vi "timing_code.vi"   [LabVIEW 2017]
uses:
  <vilib>/myRIO/Common/Instrument Driver Framework/myRIO v1.0/DIO/typedefs/DIO Channels Enum.ctl
  <vilib>/myRIO/Common/Instrument Driver Framework/myRIO v1.0/DIO/typedefs/DIO Channels List.ctl
  <vilib>/myRIO/Common/Instrument Driver Framework/Utilities/typedefs/Generic FPGA Reference.ctl
  <vilib>/myRIO/Common/Instrument Driver Framework/Utilities/typedefs/myRIO v1.0 Reference.ctl
  <vilib>/myRIO/Common/Instrument Driver Framework/Utilities/typedefs/Hardware Version Enum.ctl
  <vilib>/myRIO/Common/Instrument Driver Framework/Utilities/typedefs/myRIO Generic Hardware Reference.ctl
  <vilib>/myRIO/Instrument Drivers/Onboard IO/DIO/typedefs/DIO Reference.ctl
  <vilib>/myRIO/Instrument Drivers/Onboard IO/DIO/DIO.lvlib
  <vilib>/myRIO/Instrument Drivers/Onboard IO/DIO/vis/Write.vi
  <vilib>/userdefined/High Color/nirio_resource_hc.ctl
  <vilib>/myRIO/Common/Instrument Driver Framework/myRIO v1.0/DIO/vis/myRIO v1.1 Open DIO.vi
  <vilib>/myRIO/Instrument Drivers/Onboard IO/DIO/vis/myRIO DIO Open.xnode
  <vilib>/myRIO/Common/Instrument Driver Framework/Utilities/vis/Is FPGA Ref Available.vi
  <vilib>/myRIO/Express VI/Onboard IO/DO/DO Express VI.xnode
types:
  T1 = typedef "DIO.lvlib/DIO Reference.ctl" = cluster{"myRIO Reference":T2, "DIO Channels List":T6}
  T2 = typedef "myRIO Generic Hardware Reference.ctl" = cluster{"myRIO Model":T3, "myRIO Hardware Reference":T4}
  T3 = typedef "Hardware Version Enum.ctl" = enum16{"Unknown", "myRIO-1900", "myRIO-1950", "roboRIO", "NI ELVIS RIO CM"}
  T4 = typedef "myRIO v1.0 Reference.ctl" = cluster{"Generic FPGA Reference":T5, "Allow multiple opens":bool}
  T5 = typedef "Generic FPGA Reference.ctl" = refnum<k20>
  T6 = typedef "DIO Channels List.ctl" = T7[]
  T7 = typedef "DIO Channels Enum.ctl" = enum16{"Not Connected", "C/DIO0", "C/DIO1", "C/DIO2", "C/DIO3", "C/DIO4", "C/DIO5", "C/DIO6", "C/DIO7", "A/DIO0", "A/DIO1", "A/DIO2", "A/DIO3", "A/DIO4", "A/DIO5", "A/DIO6", "A/DIO7", "A/DIO8", "A/DIO9", "A/DIO10", "A/DIO11", "A/DIO12", "A/DIO13", "A/DIO14", "A/DIO15", "B/DIO0", "B/DIO1", "B/DIO2", "B/DIO3", "B/DIO4", "B/DIO5", "B/DIO6", "B/DIO7", "B/DIO8", "B/DIO9", "B/DIO10", "B/DIO11", "B/DIO12", "B/DIO13", "B/DIO14", "B/DIO15", "LED0", "LED1", "LED2", "LED3", "Button0", "DIO/DIO0", "DIO/DIO1", "DIO/DIO2", "DIO/DIO3", "DIO/DIO4", "DIO/DIO5", "DIO/DIO6", "DIO/DIO7", "DIO/DIO8", "DIO/DIO9", "SPI/CS0", "SPI/CS1", "SPI/CS2", "SPI/CS3", "LED RADIO (Green)", "LED RADIO (Red)", "LED COMM (Green)", "LED COMM (Red)", "LED MODE (Green)", "LED MODE (Red)"}
  T8 = typedef "nirio_resource_hc.ctl" = tag
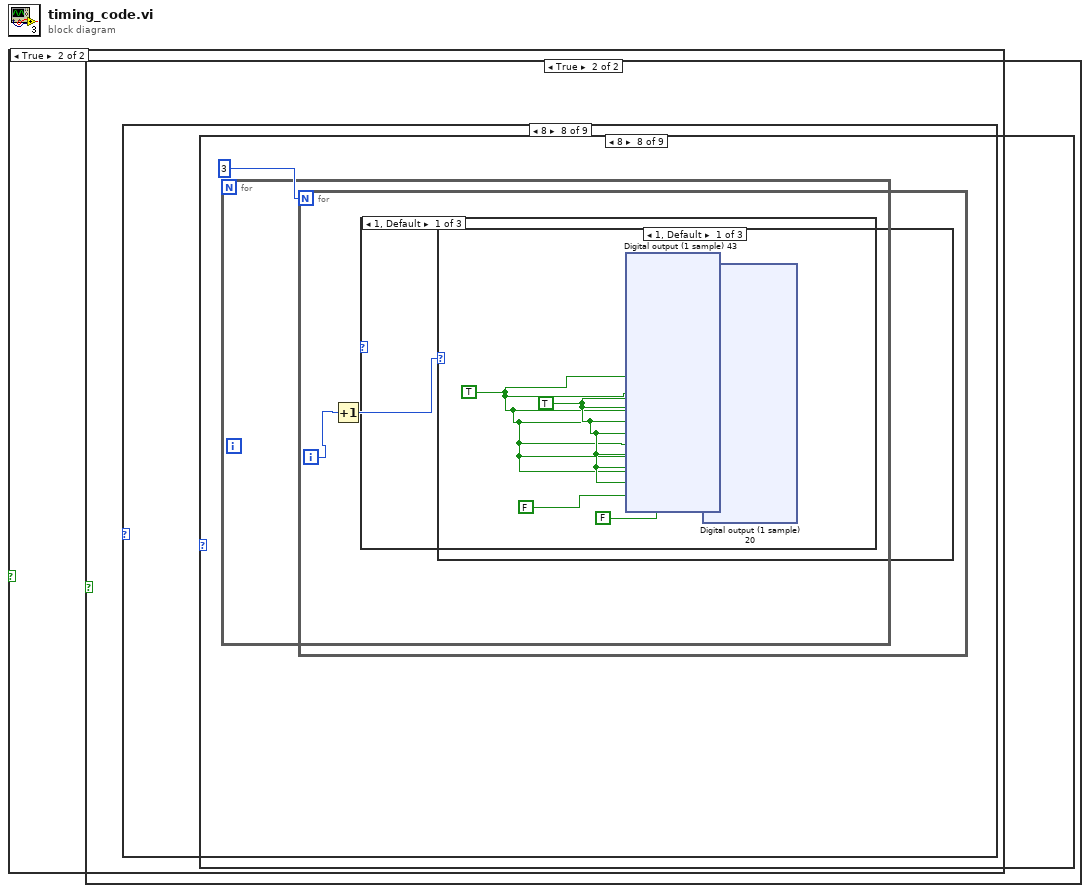
[diagram p0: block diagram]
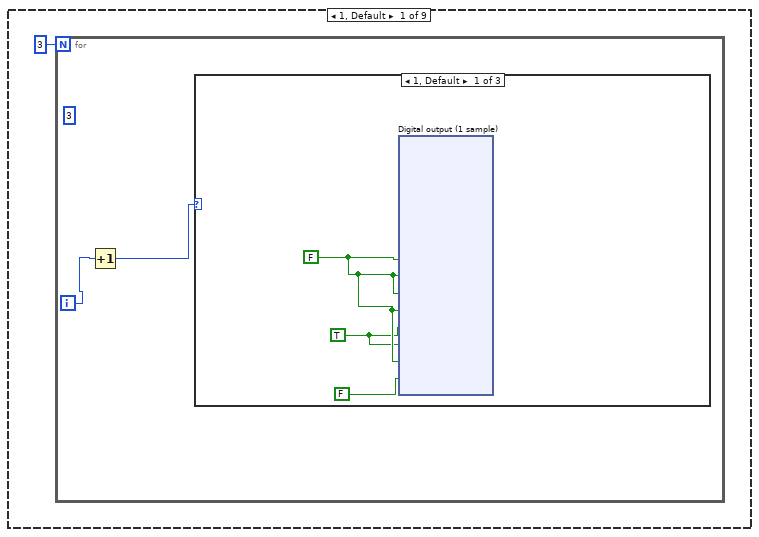
[diagram p3: hidden frame]
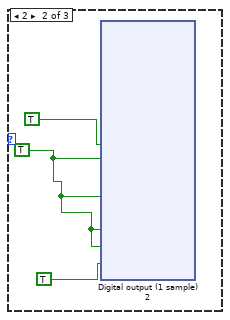
[diagram p4: hidden frame]
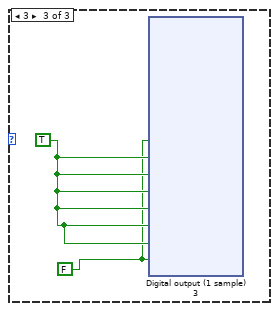
[diagram p5: hidden frame]
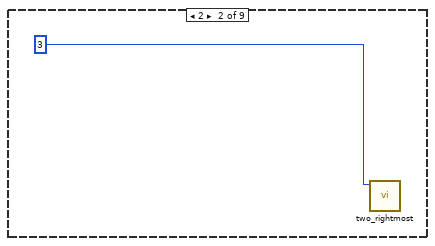
[diagram p6: hidden frame]
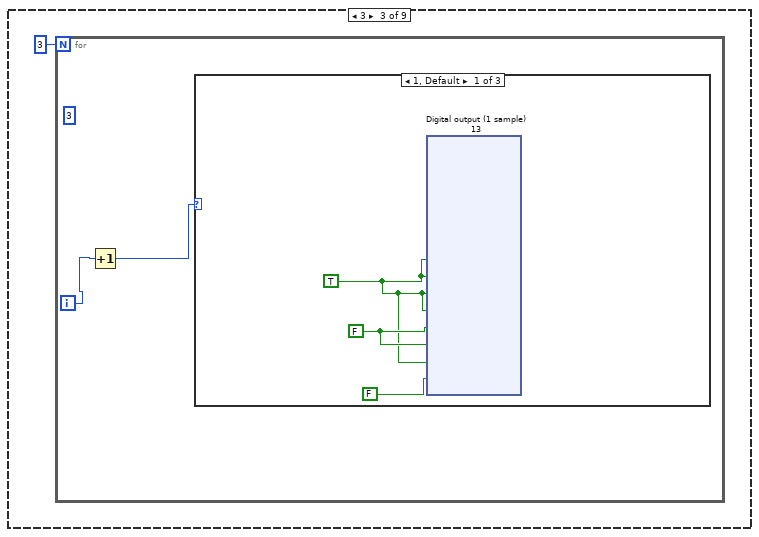
[diagram p7: hidden frame]
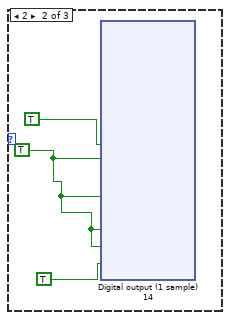
[diagram p8: hidden frame]
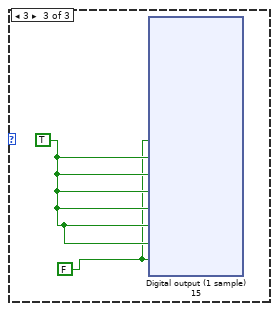
[diagram p9: hidden frame]
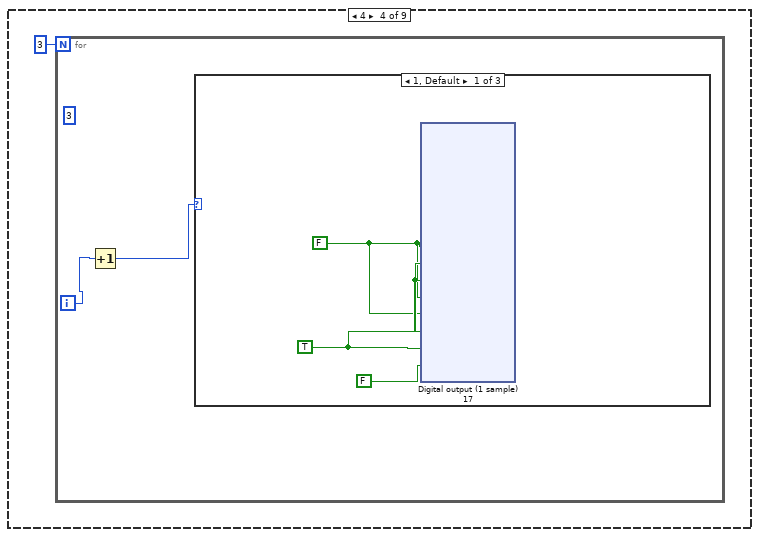
[diagram p10: hidden frame]
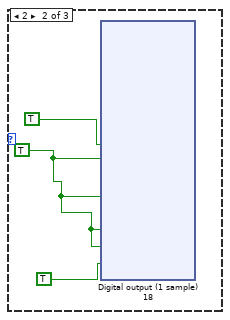
[diagram p11: hidden frame]
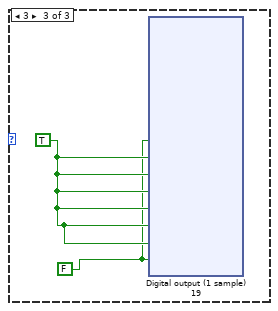
[diagram p12: hidden frame]
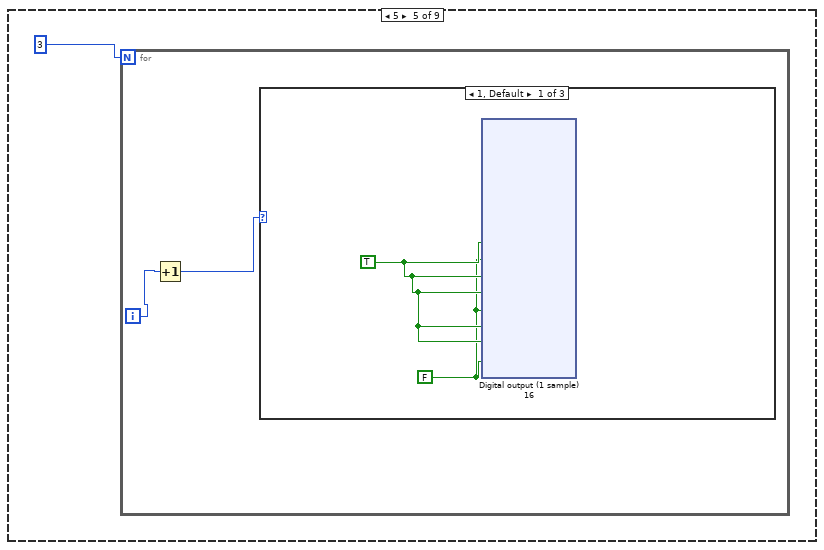
[diagram p13: hidden frame]
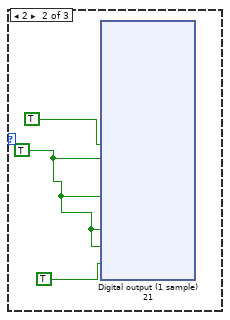
[diagram p14: hidden frame]
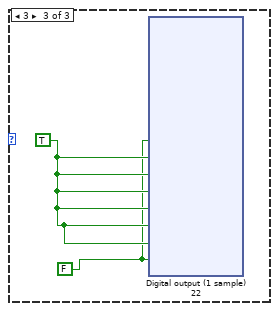
[diagram p15: hidden frame]
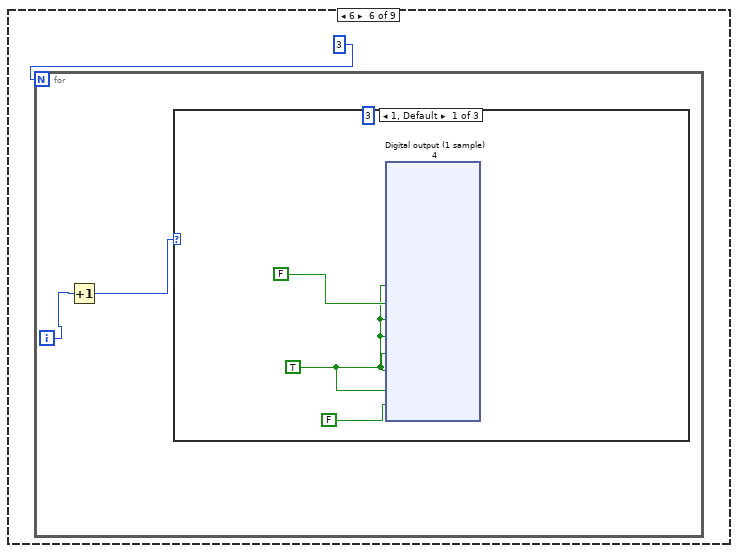
[diagram p16: hidden frame]
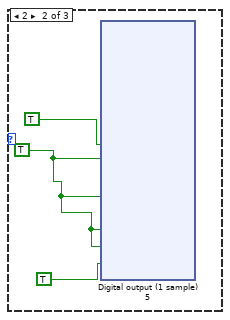
[diagram p17: hidden frame]
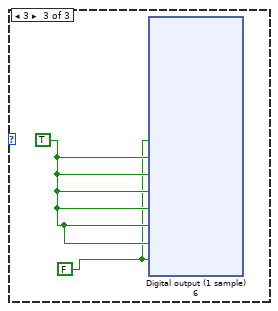
[diagram p18: hidden frame]
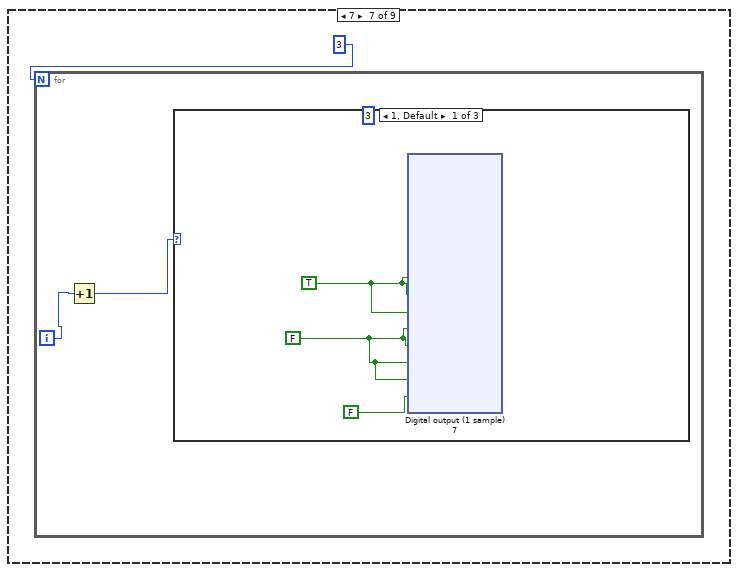
[diagram p19: hidden frame]
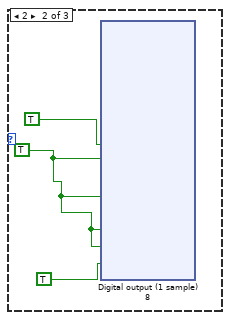
[diagram p20: hidden frame]
diagram:
  n1 = case shown="True" {
    selector: _ -> [_ _]
    frame False {
    }
    frame True {
      n2 = case shown="8" {
        selector: _ -> [_ _ _ _ _ _ _ _ _]
        frame 1, Default {
          (unwired) 3
          n3 = for {
            N: 3 -> [_]
            i -> [w3]
            n4 = Increment(x=w3) -> (x+1=w2:i32)
            n5 = case shown="1, Default" w2 {
              frame 1, Default {
                w4 = TRUE
                w5 = FALSE
                n6 = xnode "Digital output (1 sample)"("A/DIO0 (Pin 11)"=w5, "A/DIO1 (Pin 13)"=w5, "A/DIO2 (Pin 15)"=w5, "A/DIO3 (Pin 17)"=w5, "A/DIO4 (Pin 19)"=w4, "A/DIO5 (Pin 21)"=w4, "A/DIO6 (Pin 23)"=w5, "A/DIO7 (Pin 25)"=FALSE) -> ()  [unwired: 1 in, 1 out]
              }
              frame 2 {
                w49 = TRUE
                n7 = xnode "Digital output (1 sample) 2"("A/DIO0 (Pin 11)"=TRUE, "A/DIO1 (Pin 13)"=w49, "A/DIO2 (Pin 15)"=w49, "A/DIO3 (Pin 17)"=w49, "A/DIO4 (Pin 19)"=w49, "A/DIO5 (Pin 21)"=w49, "A/DIO6 (Pin 23)"=w49, "A/DIO7 (Pin 25)"=TRUE) -> ()  [unwired: 1 in, 1 out]
              }
              frame 3 {
                w95 = TRUE
                w94 = FALSE
                n8 = xnode "Digital output (1 sample) 3"("A/DIO0 (Pin 11)"=w94, "A/DIO1 (Pin 13)"=w95, "A/DIO2 (Pin 15)"=w95, "A/DIO3 (Pin 17)"=w95, "A/DIO4 (Pin 19)"=w95, "A/DIO5 (Pin 21)"=w95, "A/DIO6 (Pin 23)"=w95, "A/DIO7 (Pin 25)"=w94) -> ()  [unwired: 1 in, 1 out]
              }
            }
          }
        }
        frame 2 {
          n9 = call "two_rightmost.vi"("Numeric"=3) -> ()  [unwired: 11 in]
        }
        frame 3 {
          (unwired) 3
          n10 = for {
            N: 3 -> [_]
            i -> [w141]
            n11 = Increment(x=w141) -> (x+1=w140:i32)
            n12 = case shown="1, Default" w140 {
              frame 1, Default {
                w143 = FALSE
                w142 = TRUE
                n13 = xnode "Digital output (1 sample) 13"("A/DIO0 (Pin 11)"=w142, "A/DIO1 (Pin 13)"=w142, "A/DIO2 (Pin 15)"=w142, "A/DIO3 (Pin 17)"=w142, "A/DIO4 (Pin 19)"=w143, "A/DIO5 (Pin 21)"=w143, "A/DIO6 (Pin 23)"=w142, "A/DIO7 (Pin 25)"=FALSE) -> ()  [unwired: 1 in, 1 out]
              }
              frame 2 {
                w187 = TRUE
                n14 = xnode "Digital output (1 sample) 14"("A/DIO0 (Pin 11)"=TRUE, "A/DIO1 (Pin 13)"=w187, "A/DIO2 (Pin 15)"=w187, "A/DIO3 (Pin 17)"=w187, "A/DIO4 (Pin 19)"=w187, "A/DIO5 (Pin 21)"=w187, "A/DIO6 (Pin 23)"=w187, "A/DIO7 (Pin 25)"=TRUE) -> ()  [unwired: 1 in, 1 out]
              }
              frame 3 {
                w233 = TRUE
                w232 = FALSE
                n15 = xnode "Digital output (1 sample) 15"("A/DIO0 (Pin 11)"=w232, "A/DIO1 (Pin 13)"=w233, "A/DIO2 (Pin 15)"=w233, "A/DIO3 (Pin 17)"=w233, "A/DIO4 (Pin 19)"=w233, "A/DIO5 (Pin 21)"=w233, "A/DIO6 (Pin 23)"=w233, "A/DIO7 (Pin 25)"=w232) -> ()  [unwired: 1 in, 1 out]
              }
            }
          }
        }
        frame 4 {
          (unwired) 3
          n16 = for {
            N: 3 -> [_]
            i -> [w278]
            n17 = Increment(x=w278) -> (x+1=w277:i32)
            n18 = case shown="1, Default" w277 {
              frame 1, Default {
                w279 = FALSE
                w280 = TRUE
                n19 = xnode "Digital output (1 sample) 17"("A/DIO0 (Pin 11)"=w279, "A/DIO1 (Pin 13)"=w280, "A/DIO2 (Pin 15)"=w280, "A/DIO3 (Pin 17)"=w279, "A/DIO4 (Pin 19)"=w279, "A/DIO5 (Pin 21)"=w280, "A/DIO6 (Pin 23)"=w280, "A/DIO7 (Pin 25)"=FALSE) -> ()  [unwired: 1 in, 1 out]
              }
              frame 2 {
                w324 = TRUE
                n20 = xnode "Digital output (1 sample) 18"("A/DIO0 (Pin 11)"=TRUE, "A/DIO1 (Pin 13)"=w324, "A/DIO2 (Pin 15)"=w324, "A/DIO3 (Pin 17)"=w324, "A/DIO4 (Pin 19)"=w324, "A/DIO5 (Pin 21)"=w324, "A/DIO6 (Pin 23)"=w324, "A/DIO7 (Pin 25)"=TRUE) -> ()  [unwired: 1 in, 1 out]
              }
              frame 3 {
                w370 = TRUE
                w369 = FALSE
                n21 = xnode "Digital output (1 sample) 19"("A/DIO0 (Pin 11)"=w369, "A/DIO1 (Pin 13)"=w370, "A/DIO2 (Pin 15)"=w370, "A/DIO3 (Pin 17)"=w370, "A/DIO4 (Pin 19)"=w370, "A/DIO5 (Pin 21)"=w370, "A/DIO6 (Pin 23)"=w370, "A/DIO7 (Pin 25)"=w369) -> ()  [unwired: 1 in, 1 out]
              }
            }
          }
        }
        frame 5 {
          n22 = for {
            N: 3 -> [_]
            i -> [w415]
            n23 = Increment(x=w415) -> (x+1=w414:i32)
            n24 = case shown="1, Default" w414 {
              frame 1, Default {
                w417 = TRUE
                w416 = FALSE
                n25 = xnode "Digital output (1 sample) 16"("A/DIO0 (Pin 11)"=w417, "A/DIO1 (Pin 13)"=w416, "A/DIO2 (Pin 15)"=w417, "A/DIO3 (Pin 17)"=w417, "A/DIO4 (Pin 19)"=w416, "A/DIO5 (Pin 21)"=w417, "A/DIO6 (Pin 23)"=w417, "A/DIO7 (Pin 25)"=w416) -> ()  [unwired: 1 in, 1 out]
              }
              frame 2 {
                w460 = TRUE
                n26 = xnode "Digital output (1 sample) 21"("A/DIO0 (Pin 11)"=TRUE, "A/DIO1 (Pin 13)"=w460, "A/DIO2 (Pin 15)"=w460, "A/DIO3 (Pin 17)"=w460, "A/DIO4 (Pin 19)"=w460, "A/DIO5 (Pin 21)"=w460, "A/DIO6 (Pin 23)"=w460, "A/DIO7 (Pin 25)"=TRUE) -> ()  [unwired: 1 in, 1 out]
              }
              frame 3 {
                w506 = TRUE
                w505 = FALSE
                n27 = xnode "Digital output (1 sample) 22"("A/DIO0 (Pin 11)"=w505, "A/DIO1 (Pin 13)"=w506, "A/DIO2 (Pin 15)"=w506, "A/DIO3 (Pin 17)"=w506, "A/DIO4 (Pin 19)"=w506, "A/DIO5 (Pin 21)"=w506, "A/DIO6 (Pin 23)"=w506, "A/DIO7 (Pin 25)"=w505) -> ()  [unwired: 1 in, 1 out]
              }
            }
          }
        }
        frame 6 {
          (unwired) 3
          n28 = for {
            N: 3 -> [_]
            i -> [w551]
            n29 = Increment(x=w551) -> (x+1=w550:i32)
            n30 = case shown="1, Default" w550 {
              frame 1, Default {
                w552 = TRUE
                n31 = xnode "Digital output (1 sample) 4"("A/DIO0 (Pin 11)"=w552, "A/DIO1 (Pin 13)"=FALSE, "A/DIO2 (Pin 15)"=w552, "A/DIO3 (Pin 17)"=w552, "A/DIO4 (Pin 19)"=w552, "A/DIO5 (Pin 21)"=w552, "A/DIO6 (Pin 23)"=w552, "A/DIO7 (Pin 25)"=FALSE) -> ()  [unwired: 1 in, 1 out]
              }
              frame 2 {
                w597 = TRUE
                n32 = xnode "Digital output (1 sample) 5"("A/DIO0 (Pin 11)"=TRUE, "A/DIO1 (Pin 13)"=w597, "A/DIO2 (Pin 15)"=w597, "A/DIO3 (Pin 17)"=w597, "A/DIO4 (Pin 19)"=w597, "A/DIO5 (Pin 21)"=w597, "A/DIO6 (Pin 23)"=w597, "A/DIO7 (Pin 25)"=TRUE) -> ()  [unwired: 1 in, 1 out]
              }
              frame 3 {
                w643 = TRUE
                w642 = FALSE
                n33 = xnode "Digital output (1 sample) 6"("A/DIO0 (Pin 11)"=w642, "A/DIO1 (Pin 13)"=w643, "A/DIO2 (Pin 15)"=w643, "A/DIO3 (Pin 17)"=w643, "A/DIO4 (Pin 19)"=w643, "A/DIO5 (Pin 21)"=w643, "A/DIO6 (Pin 23)"=w643, "A/DIO7 (Pin 25)"=w642) -> ()  [unwired: 1 in, 1 out]
              }
            }
          }
        }
        frame 7 {
          (unwired) 3
          n34 = for {
            N: 3 -> [_]
            i -> [w688]
            n35 = Increment(x=w688) -> (x+1=w687:i32)
            n36 = case shown="1, Default" w687 {
              frame 1, Default {
                w689 = FALSE
                w690 = TRUE
                n37 = xnode "Digital output (1 sample) 7"("A/DIO0 (Pin 11)"=w690, "A/DIO1 (Pin 13)"=w690, "A/DIO2 (Pin 15)"=w690, "A/DIO3 (Pin 17)"=w689, "A/DIO4 (Pin 19)"=w689, "A/DIO5 (Pin 21)"=w689, "A/DIO6 (Pin 23)"=w689, "A/DIO7 (Pin 25)"=FALSE) -> ()  [unwired: 1 in, 1 out]
              }
              frame 2 {
                w734 = TRUE
                n38 = xnode "Digital output (1 sample) 8"("A/DIO0 (Pin 11)"=TRUE, "A/DIO1 (Pin 13)"=w734, "A/DIO2 (Pin 15)"=w734, "A/DIO3 (Pin 17)"=w734, "A/DIO4 (Pin 19)"=w734, "A/DIO5 (Pin 21)"=w734, "A/DIO6 (Pin 23)"=w734, "A/DIO7 (Pin 25)"=TRUE) -> ()  [unwired: 1 in, 1 out]
              }
              frame 3 {
                w780 = TRUE
                w779 = FALSE
                n39 = xnode "Digital output (1 sample) 9"("A/DIO0 (Pin 11)"=w779, "A/DIO1 (Pin 13)"=w780, "A/DIO2 (Pin 15)"=w780, "A/DIO3 (Pin 17)"=w780, "A/DIO4 (Pin 19)"=w780, "A/DIO5 (Pin 21)"=w780, "A/DIO6 (Pin 23)"=w780, "A/DIO7 (Pin 25)"=w779) -> ()  [unwired: 1 in, 1 out]
              }
            }
          }
        }
        frame 8 {
          n40 = for {
            N: 3 -> [_]
            i -> [w825]
            n41 = Increment(x=w825) -> (x+1=w824:i32)
            n42 = case shown="1, Default" w824 {
              frame 1, Default {
                w826 = TRUE
                n43 = case shown="True" {
                  selector: _ -> [_ _]
                  frame False {
                  }
                  frame True {
                    n44 = case shown="8" {
                      selector: _ -> [_ _ _ _ _ _ _ _ _]
                      frame 1, Default {
                        (unwired) 3
                        n45 = for {
                          N: 3 -> [_]
                          i -> [w830]
                          n46 = Increment(x=w830) -> (x+1=w829:i32)
                          n47 = case shown="1, Default" w829 {
                            frame 1, Default {
                              w831 = TRUE
                              w832 = FALSE
                              n48 = xnode "Digital output (1 sample) 25"("A/DIO0 (Pin 11)"=w832, "A/DIO1 (Pin 13)"=w832, "A/DIO2 (Pin 15)"=w832, "A/DIO3 (Pin 17)"=w832, "A/DIO4 (Pin 19)"=w831, "A/DIO5 (Pin 21)"=w831, "A/DIO6 (Pin 23)"=w832, "A/DIO7 (Pin 25)"=FALSE) -> ()  [unwired: 1 in, 1 out]
                            }
                            frame 2 {
                              w876 = TRUE
                              n49 = xnode "Digital output (1 sample) 26"("A/DIO0 (Pin 11)"=TRUE, "A/DIO1 (Pin 13)"=w876, "A/DIO2 (Pin 15)"=w876, "A/DIO3 (Pin 17)"=w876, "A/DIO4 (Pin 19)"=w876, "A/DIO5 (Pin 21)"=w876, "A/DIO6 (Pin 23)"=w876, "A/DIO7 (Pin 25)"=TRUE) -> ()  [unwired: 1 in, 1 out]
                            }
                            frame 3 {
                              w922 = TRUE
                              w921 = FALSE
                              n50 = xnode "Digital output (1 sample) 27"("A/DIO0 (Pin 11)"=w921, "A/DIO1 (Pin 13)"=w922, "A/DIO2 (Pin 15)"=w922, "A/DIO3 (Pin 17)"=w922, "A/DIO4 (Pin 19)"=w922, "A/DIO5 (Pin 21)"=w922, "A/DIO6 (Pin 23)"=w922, "A/DIO7 (Pin 25)"=w921) -> ()  [unwired: 1 in, 1 out]
                            }
                          }
                        }
                      }
                      frame 2 {
                        n51 = call "two_rightmost.vi"("Numeric"=3) -> ()  [unwired: 11 in]
                      }
                      frame 3 {
                        (unwired) 3
                        n52 = for {
                          N: 3 -> [_]
                          i -> [w968]
                          n53 = Increment(x=w968) -> (x+1=w967:i32)
                          n54 = case shown="1, Default" w967 {
                            frame 1, Default {
                              w970 = FALSE
                              w969 = TRUE
                              n55 = xnode "Digital output (1 sample) 28"("A/DIO0 (Pin 11)"=w969, "A/DIO1 (Pin 13)"=w969, "A/DIO2 (Pin 15)"=w969, "A/DIO3 (Pin 17)"=w969, "A/DIO4 (Pin 19)"=w970, "A/DIO5 (Pin 21)"=w970, "A/DIO6 (Pin 23)"=w969, "A/DIO7 (Pin 25)"=FALSE) -> ()  [unwired: 1 in, 1 out]
                            }
                            frame 2 {
                              w1014 = TRUE
                              n56 = xnode "Digital output (1 sample) 29"("A/DIO0 (Pin 11)"=TRUE, "A/DIO1 (Pin 13)"=w1014, "A/DIO2 (Pin 15)"=w1014, "A/DIO3 (Pin 17)"=w1014, "A/DIO4 (Pin 19)"=w1014, "A/DIO5 (Pin 21)"=w1014, "A/DIO6 (Pin 23)"=w1014, "A/DIO7 (Pin 25)"=TRUE) -> ()  [unwired: 1 in, 1 out]
                            }
                            frame 3 {
                              w1060 = TRUE
                              w1059 = FALSE
                              n57 = xnode "Digital output (1 sample) 30"("A/DIO0 (Pin 11)"=w1059, "A/DIO1 (Pin 13)"=w1060, "A/DIO2 (Pin 15)"=w1060, "A/DIO3 (Pin 17)"=w1060, "A/DIO4 (Pin 19)"=w1060, "A/DIO5 (Pin 21)"=w1060, "A/DIO6 (Pin 23)"=w1060, "A/DIO7 (Pin 25)"=w1059) -> ()  [unwired: 1 in, 1 out]
                            }
                          }
                        }
                      }
                      frame 4 {
                        (unwired) 3
                        n58 = for {
                          N: 3 -> [_]
                          i -> [w1105]
                          n59 = Increment(x=w1105) -> (x+1=w1104:i32)
                          n60 = case shown="1, Default" w1104 {
                            frame 1, Default {
                              w1106 = FALSE
                              w1107 = TRUE
                              n61 = xnode "Digital output (1 sample) 31"("A/DIO0 (Pin 11)"=w1106, "A/DIO1 (Pin 13)"=w1107, "A/DIO2 (Pin 15)"=w1107, "A/DIO3 (Pin 17)"=w1106, "A/DIO4 (Pin 19)"=w1106, "A/DIO5 (Pin 21)"=w1107, "A/DIO6 (Pin 23)"=w1107, "A/DIO7 (Pin 25)"=FALSE) -> ()  [unwired: 1 in, 1 out]
                            }
                            frame 2 {
                              w1151 = TRUE
                              n62 = xnode "Digital output (1 sample) 32"("A/DIO0 (Pin 11)"=TRUE, "A/DIO1 (Pin 13)"=w1151, "A/DIO2 (Pin 15)"=w1151, "A/DIO3 (Pin 17)"=w1151, "A/DIO4 (Pin 19)"=w1151, "A/DIO5 (Pin 21)"=w1151, "A/DIO6 (Pin 23)"=w1151, "A/DIO7 (Pin 25)"=TRUE) -> ()  [unwired: 1 in, 1 out]
                            }
                            frame 3 {
                              w1197 = TRUE
                              w1196 = FALSE
                              n63 = xnode "Digital output (1 sample) 33"("A/DIO0 (Pin 11)"=w1196, "A/DIO1 (Pin 13)"=w1197, "A/DIO2 (Pin 15)"=w1197, "A/DIO3 (Pin 17)"=w1197, "A/DIO4 (Pin 19)"=w1197, "A/DIO5 (Pin 21)"=w1197, "A/DIO6 (Pin 23)"=w1197, "A/DIO7 (Pin 25)"=w1196) -> ()  [unwired: 1 in, 1 out]
                            }
                          }
                        }
                      }
                      frame 5 {
                        n64 = for {
                          N: 3 -> [_]
                          i -> [w1242]
                          n65 = Increment(x=w1242) -> (x+1=w1241:i32)
                          n66 = case shown="1, Default" w1241 {
                            frame 1, Default {
                              w1244 = TRUE
                              w1243 = FALSE
                              n67 = xnode "Digital output (1 sample) 34"("A/DIO0 (Pin 11)"=w1244, "A/DIO1 (Pin 13)"=w1243, "A/DIO2 (Pin 15)"=w1244, "A/DIO3 (Pin 17)"=w1244, "A/DIO4 (Pin 19)"=w1243, "A/DIO5 (Pin 21)"=w1244, "A/DIO6 (Pin 23)"=w1244, "A/DIO7 (Pin 25)"=w1243) -> ()  [unwired: 1 in, 1 out]
                            }
                            frame 2 {
                              w1287 = TRUE
                              n68 = xnode "Digital output (1 sample) 35"("A/DIO0 (Pin 11)"=TRUE, "A/DIO1 (Pin 13)"=w1287, "A/DIO2 (Pin 15)"=w1287, "A/DIO3 (Pin 17)"=w1287, "A/DIO4 (Pin 19)"=w1287, "A/DIO5 (Pin 21)"=w1287, "A/DIO6 (Pin 23)"=w1287, "A/DIO7 (Pin 25)"=TRUE) -> ()  [unwired: 1 in, 1 out]
                            }
                            frame 3 {
                              w1333 = TRUE
                              w1332 = FALSE
                              n69 = xnode "Digital output (1 sample) 36"("A/DIO0 (Pin 11)"=w1332, "A/DIO1 (Pin 13)"=w1333, "A/DIO2 (Pin 15)"=w1333, "A/DIO3 (Pin 17)"=w1333, "A/DIO4 (Pin 19)"=w1333, "A/DIO5 (Pin 21)"=w1333, "A/DIO6 (Pin 23)"=w1333, "A/DIO7 (Pin 25)"=w1332) -> ()  [unwired: 1 in, 1 out]
                            }
                          }
                        }
                      }
                      frame 6 {
                        (unwired) 3
                        n70 = for {
                          N: 3 -> [_]
                          i -> [w1378]
                          n71 = Increment(x=w1378) -> (x+1=w1377:i32)
                          n72 = case shown="1, Default" w1377 {
                            frame 1, Default {
                              w1379 = TRUE
                              n73 = xnode "Digital output (1 sample) 37"("A/DIO0 (Pin 11)"=w1379, "A/DIO1 (Pin 13)"=FALSE, "A/DIO2 (Pin 15)"=w1379, "A/DIO3 (Pin 17)"=w1379, "A/DIO4 (Pin 19)"=w1379, "A/DIO5 (Pin 21)"=w1379, "A/DIO6 (Pin 23)"=w1379, "A/DIO7 (Pin 25)"=FALSE) -> ()  [unwired: 1 in, 1 out]
                            }
                            frame 2 {
                              w1424 = TRUE
                              n74 = xnode "Digital output (1 sample) 38"("A/DIO0 (Pin 11)"=TRUE, "A/DIO1 (Pin 13)"=w1424, "A/DIO2 (Pin 15)"=w1424, "A/DIO3 (Pin 17)"=w1424, "A/DIO4 (Pin 19)"=w1424, "A/DIO5 (Pin 21)"=w1424, "A/DIO6 (Pin 23)"=w1424, "A/DIO7 (Pin 25)"=TRUE) -> ()  [unwired: 1 in, 1 out]
                            }
                            frame 3 {
                              w1470 = TRUE
                              w1469 = FALSE
                              n75 = xnode "Digital output (1 sample) 39"("A/DIO0 (Pin 11)"=w1469, "A/DIO1 (Pin 13)"=w1470, "A/DIO2 (Pin 15)"=w1470, "A/DIO3 (Pin 17)"=w1470, "A/DIO4 (Pin 19)"=w1470, "A/DIO5 (Pin 21)"=w1470, "A/DIO6 (Pin 23)"=w1470, "A/DIO7 (Pin 25)"=w1469) -> ()  [unwired: 1 in, 1 out]
                            }
                          }
                        }
                      }
                      frame 7 {
                        (unwired) 3
                        n76 = for {
                          N: 3 -> [_]
                          i -> [w1515]
                          n77 = Increment(x=w1515) -> (x+1=w1514:i32)
                          n78 = case shown="1, Default" w1514 {
                            frame 1, Default {
                              w1516 = FALSE
                              w1517 = TRUE
                              n79 = xnode "Digital output (1 sample) 40"("A/DIO0 (Pin 11)"=w1517, "A/DIO1 (Pin 13)"=w1517, "A/DIO2 (Pin 15)"=w1517, "A/DIO3 (Pin 17)"=w1516, "A/DIO4 (Pin 19)"=w1516, "A/DIO5 (Pin 21)"=w1516, "A/DIO6 (Pin 23)"=w1516, "A/DIO7 (Pin 25)"=FALSE) -> ()  [unwired: 1 in, 1 out]
                            }
                            frame 2 {
                              w1561 = TRUE
                              n80 = xnode "Digital output (1 sample) 41"("A/DIO0 (Pin 11)"=TRUE, "A/DIO1 (Pin 13)"=w1561, "A/DIO2 (Pin 15)"=w1561, "A/DIO3 (Pin 17)"=w1561, "A/DIO4 (Pin 19)"=w1561, "A/DIO5 (Pin 21)"=w1561, "A/DIO6 (Pin 23)"=w1561, "A/DIO7 (Pin 25)"=TRUE) -> ()  [unwired: 1 in, 1 out]
                            }
                            frame 3 {
                              w1607 = TRUE
                              w1606 = FALSE
                              n81 = xnode "Digital output (1 sample) 42"("A/DIO0 (Pin 11)"=w1606, "A/DIO1 (Pin 13)"=w1607, "A/DIO2 (Pin 15)"=w1607, "A/DIO3 (Pin 17)"=w1607, "A/DIO4 (Pin 19)"=w1607, "A/DIO5 (Pin 21)"=w1607, "A/DIO6 (Pin 23)"=w1607, "A/DIO7 (Pin 25)"=w1606) -> ()  [unwired: 1 in, 1 out]
                            }
                          }
                        }
                      }
                      frame 8 {
                        n82 = for {
                          N: 3 -> [_]
                          i -> [w1652]
                          n83 = Increment(x=w1652) -> (x+1=w1651:i32)
                          n84 = case shown="1, Default" w1651 {
                            frame 1, Default {
                              w1653 = TRUE
                              n85 = xnode "Digital output (1 sample) 43"("A/DIO0 (Pin 11)"=w1653, "A/DIO1 (Pin 13)"=w1653, "A/DIO2 (Pin 15)"=w1653, "A/DIO3 (Pin 17)"=w1653, "A/DIO4 (Pin 19)"=w1653, "A/DIO5 (Pin 21)"=w1653, "A/DIO6 (Pin 23)"=w1653, "A/DIO7 (Pin 25)"=FALSE) -> ()  [unwired: 1 in, 1 out]
                            }
                            frame 2 {
                              w1697 = TRUE
                              n86 = xnode "Digital output (1 sample) 44"("A/DIO0 (Pin 11)"=TRUE, "A/DIO1 (Pin 13)"=w1697, "A/DIO2 (Pin 15)"=w1697, "A/DIO3 (Pin 17)"=w1697, "A/DIO4 (Pin 19)"=w1697, "A/DIO5 (Pin 21)"=w1697, "A/DIO6 (Pin 23)"=w1697, "A/DIO7 (Pin 25)"=TRUE) -> ()  [unwired: 1 in, 1 out]
                            }
                            frame 3 {
                              w1743 = TRUE
                              w1742 = FALSE
                              n87 = xnode "Digital output (1 sample) 45"("A/DIO0 (Pin 11)"=w1742, "A/DIO1 (Pin 13)"=w1743, "A/DIO2 (Pin 15)"=w1743, "A/DIO3 (Pin 17)"=w1743, "A/DIO4 (Pin 19)"=w1743, "A/DIO5 (Pin 21)"=w1743, "A/DIO6 (Pin 23)"=w1743, "A/DIO7 (Pin 25)"=w1742) -> ()  [unwired: 1 in, 1 out]
                            }
                          }
                        }
                      }
                      frame 9 {
                        (unwired) 3
                        n88 = for {
                          N: 3 -> [_]
                          i -> [w1788]
                          n89 = Increment(x=w1788) -> (x+1=w1787:i32)
                          n90 = case shown="1, Default" w1787 {
                            frame 1, Default {
                              w1789 = TRUE
                              w1790 = FALSE
                              n91 = xnode "Digital output (1 sample) 46"("A/DIO0 (Pin 11)"=w1789, "A/DIO1 (Pin 13)"=w1789, "A/DIO2 (Pin 15)"=w1789, "A/DIO3 (Pin 17)"=w1790, "A/DIO4 (Pin 19)"=w1790, "A/DIO5 (Pin 21)"=w1789, "A/DIO6 (Pin 23)"=w1789, "A/DIO7 (Pin 25)"=w1790) -> ()  [unwired: 1 in, 1 out]
                            }
                            frame 2 {
                              w1833 = TRUE
                              n92 = xnode "Digital output (1 sample) 47"("A/DIO0 (Pin 11)"=TRUE, "A/DIO1 (Pin 13)"=w1833, "A/DIO2 (Pin 15)"=w1833, "A/DIO3 (Pin 17)"=w1833, "A/DIO4 (Pin 19)"=w1833, "A/DIO5 (Pin 21)"=w1833, "A/DIO6 (Pin 23)"=w1833, "A/DIO7 (Pin 25)"=TRUE) -> ()  [unwired: 1 in, 1 out]
                            }
                            frame 3 {
                              w1879 = TRUE
                              w1878 = FALSE
                              n93 = xnode "Digital output (1 sample) 48"("A/DIO0 (Pin 11)"=w1878, "A/DIO1 (Pin 13)"=w1879, "A/DIO2 (Pin 15)"=w1879, "A/DIO3 (Pin 17)"=w1879, "A/DIO4 (Pin 19)"=w1879, "A/DIO5 (Pin 21)"=w1879, "A/DIO6 (Pin 23)"=w1879, "A/DIO7 (Pin 25)"=w1878) -> ()  [unwired: 1 in, 1 out]
                            }
                          }
                        }
                      }
                    }
                  }
                }
                n94 = xnode "Digital output (1 sample) 20"("A/DIO0 (Pin 11)"=w826, "A/DIO1 (Pin 13)"=w826, "A/DIO2 (Pin 15)"=w826, "A/DIO3 (Pin 17)"=w826, "A/DIO4 (Pin 19)"=w826, "A/DIO5 (Pin 21)"=w826, "A/DIO6 (Pin 23)"=w826, "A/DIO7 (Pin 25)"=FALSE) -> ()  [unwired: 1 in, 1 out]
              }
              frame 2 {
                w1964 = TRUE
                n95 = xnode "Digital output (1 sample) 23"("A/DIO0 (Pin 11)"=TRUE, "A/DIO1 (Pin 13)"=w1964, "A/DIO2 (Pin 15)"=w1964, "A/DIO3 (Pin 17)"=w1964, "A/DIO4 (Pin 19)"=w1964, "A/DIO5 (Pin 21)"=w1964, "A/DIO6 (Pin 23)"=w1964, "A/DIO7 (Pin 25)"=TRUE) -> ()  [unwired: 1 in, 1 out]
              }
              frame 3 {
                w2010 = TRUE
                w2009 = FALSE
                n96 = xnode "Digital output (1 sample) 24"("A/DIO0 (Pin 11)"=w2009, "A/DIO1 (Pin 13)"=w2010, "A/DIO2 (Pin 15)"=w2010, "A/DIO3 (Pin 17)"=w2010, "A/DIO4 (Pin 19)"=w2010, "A/DIO5 (Pin 21)"=w2010, "A/DIO6 (Pin 23)"=w2010, "A/DIO7 (Pin 25)"=w2009) -> ()  [unwired: 1 in, 1 out]
              }
            }
          }
        }
        frame 9 {
          (unwired) 3
          n97 = for {
            N: 3 -> [_]
            i -> [w2055]
            n98 = Increment(x=w2055) -> (x+1=w2054:i32)
            n99 = case shown="1, Default" w2054 {
              frame 1, Default {
                w2056 = TRUE
                w2057 = FALSE
                n100 = xnode "Digital output (1 sample) 10"("A/DIO0 (Pin 11)"=w2056, "A/DIO1 (Pin 13)"=w2056, "A/DIO2 (Pin 15)"=w2056, "A/DIO3 (Pin 17)"=w2057, "A/DIO4 (Pin 19)"=w2057, "A/DIO5 (Pin 21)"=w2056, "A/DIO6 (Pin 23)"=w2056, "A/DIO7 (Pin 25)"=w2057) -> ()  [unwired: 1 in, 1 out]
              }
              frame 2 {
                w2100 = TRUE
                n101 = xnode "Digital output (1 sample) 11"("A/DIO0 (Pin 11)"=TRUE, "A/DIO1 (Pin 13)"=w2100, "A/DIO2 (Pin 15)"=w2100, "A/DIO3 (Pin 17)"=w2100, "A/DIO4 (Pin 19)"=w2100, "A/DIO5 (Pin 21)"=w2100, "A/DIO6 (Pin 23)"=w2100, "A/DIO7 (Pin 25)"=TRUE) -> ()  [unwired: 1 in, 1 out]
              }
              frame 3 {
                w2146 = TRUE
                w2145 = FALSE
                n102 = xnode "Digital output (1 sample) 12"("A/DIO0 (Pin 11)"=w2145, "A/DIO1 (Pin 13)"=w2146, "A/DIO2 (Pin 15)"=w2146, "A/DIO3 (Pin 17)"=w2146, "A/DIO4 (Pin 19)"=w2146, "A/DIO5 (Pin 21)"=w2146, "A/DIO6 (Pin 23)"=w2146, "A/DIO7 (Pin 25)"=w2145) -> ()  [unwired: 1 in, 1 out]
              }
            }
          }
        }
      }
    }
  }
